vi "VGS Volume Project from RAW Volume.vi"() -> ()   [LabVIEW 2022 SP3, in "LV_VGS.lvlib"]
uses:
  LV_VGS.lvlib
  typedefs/3D Size (I32).ctl
  typedefs/3D Resolution (SGL).ctl
  RemoteControlClient/VGS_RemoteControlClient.lvclass
  Project/VGS_Project.lvclass
  VolumeDescriptor+File/VGS_VolumeDescriptor+File.lvclass
  VolumeDescriptor/VGS_VolumeDescriptor.lvclass
  ManufacturerInfo/VGS_ManufacturerInfo.lvclass
  ComponentInfo/VGS_ComponentInfo.lvclass
panel:
  out "Save Time, ms":u32=16563
  # "Original Volume Example rewritten in LabVIEW"
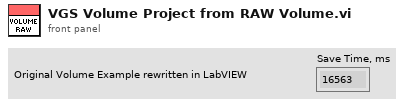
[diagram p1: front panel]
types:
  T1 = enum16{"big-endian, network order", "native, host order", "little-endian"}
  T2 = typedef "LV_VGS.lvlib/3D Resolution (SGL).ctl" = cluster{"X":sgl, "Y":sgl, "Z":sgl}
  T3 = typedef "LV_VGS.lvlib/3D Size (I32).ctl" = cluster{"X":i32, "Y":i32, "Z":i32}
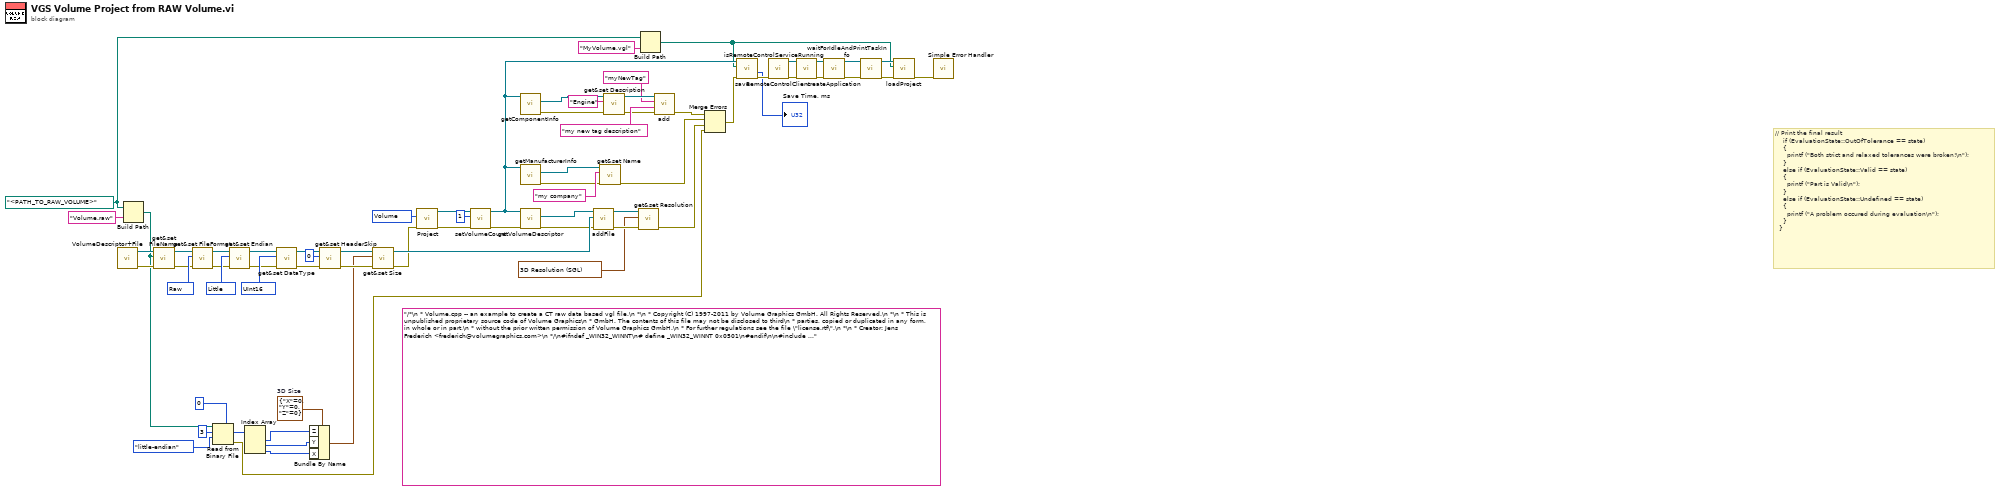
[diagram p0: block diagram]
diagram:
  w16 = 1448153088 items=["Volume"=1448153088, "Reconstruction"=1448153089] ("type")
  w7 = T3 {"X"=0, "Y"=0, "Z"=0}  # 3D Size
  w59 = 1448157378 items=["UInt8"=1448157376, "Int8"=1448157377, "UInt16"=1448157378, "Int16"=1448157379, "UInt32"=1448157380, "Int32"=1448157381, "Float"=1448157382, "Rgb8"=1448157383] ("DataType")
  w62 = 1448157440 items=["Little"=1448157440, "Big"=1448157441] ("Endian")
  w65 = 1448157312 items=["Raw"=1448157312, "Gzip"=1448157313, "Tiff"=1448157314, "Jpeg"=1448157315, "Bmp"=1448157316, "Bir"=1448157317, "Toshiba"=1448157318, "Shimadzu"=1448157319, "Pnm"=1448157320, "Jpeg2"=1448157321, "Yxlon"=1448157322, "Hdf"=1448157323, "Dicom"=1448157324, "Imtec"=1448157325, "Aracor"=1448157326, "Fhg"=1448157327] ("FileFormat")
  w18 = path "<PATH_TO_RAW_VOLUME>" ("replacementPattern")
  (unwired) "/*\n * Volume.cpp -- an example to create a CT raw data based vgl file.\n *\n * Copyright (C) 1997-2011 by Volume Graphics GmbH. All Rights Reserved.\n *\n * This is unpublished proprietary source code of Volume Graphics\n * GmbH. The contents of this file may not be disclosed to third\n * parties, copied or duplicated in any form, in whole or in part,\n * without the prior written permission of Volume Graphics GmbH.\n * For further regulations see the file \"license.rtf\".\n *\n * Creator: Jens Frederich <frederich@volumegraphics.com>\n */\n#ifndef _WIN32_WINNT\n# define _WIN32_WINNT 0x0501\n#endif\n\n#include <tchar.h>\n\n#include <vgs.project/project.h>\n\nusing namespace vgs::project;\nusing namespace vgs::project::volume;\n\nint _tmain (int argc, _TCHAR* argv[])\n{\n  Project* p = new Project (Project::Type::Volume);\n  assert (p != NULL);\n\n  // add single raw block file\n  {\n    VolumeDescriptor::File data;\n\n    data.setFileName   (\"D:/Volume Graphics/API TEST/vgs/data/engine.gz\");\n    data.setFileFormat (volume::FileFormat::Gzip);\n    data.setEndian     (volume::Endian::Little);\n    data.setDataType   (DataType::UInt8);\n    data.setHeaderSkip (0);\n    data.setSize       (Vector3<int> (256, 256, 110));\n    \n    p->setVolumeCount (1);\n    VolumeDescriptor* vd = p->getVolumeDescriptor (0);\n    assert (vd != NULL);\n\n    vd->addFile (data);\n  }\n\n  // add some meta data\n  {\n    ManufacturerInfo* mi = p->getManufacturerInfo ();\n    mi->setName (\"My company\");\n\n    ComponentInfo* ci = p->getComponentInfo ();\n    ci->setDescription (\"Engine\");\n\n    // add user defined tag\n    ci->add (\"myNewTag\", \"my new tag description\");\n\n    // add logo and preview\n    //p->setLogo    (\"c:/data/logo.png\");\n    //p->setPreview (\"c:/data/scene_preview.png\");\n  }\n\n  // create VG project\n  {\n    bool ok = true;\n\n    ok = p->save (std::string (\"D:/Volume Graphics/API TEST/vgs/data/my-first-volume1.vgl\"));\n    if (true != ok)\n    {\n      Error::ErrorCode err = Error::getLastError ();\n\t  printf(\"something is wrong, error code = %d\", err);\n      __debugbreak ();\n    }\n  }\n\n  // cleanup\n  if (p != NULL)\n  {\n    delete p;\n  }\n\n  return 0;\n}\n\n"
  # "// Print the final result\n    if (EvaluationState::OutOfTolerance == state)\n    {\n      printf (\"Both strict and relaxed tolerances were broken!\\n\");\n    }\n    else if (EvaluationState::Valid == state)\n    {\n      printf (\"Part is Valid\\n\");\n    }\n    else if (EvaluationState::Undefined == state)\n    {\n      printf (\"A problem occured during evaluation\\n\");\n    }\n  }"
  n1 = call "VolumeDescriptor+File.vi"() -> ("error out"=w67:errorcluster, "VGS_VolumeDescriptor+File out"=w69:refnum<class "VGS_VolumeDescriptor+File.lvclass">)  [unwired: 10 in]
  n2 = Build Path(base path=w18, name or relative path="Volume.raw") -> (appended path=w9:path)
  n3 = call "get&set FileName.vi"("error in (no error)"=w67, "FileName"=w9, "VGS_VolumeDescriptor+File in"=w69) -> ("error out"=w64:errorcluster, "VGS_VolumeDescriptor+File out"=w66:refnum<class "VGS_VolumeDescriptor+File.lvclass">)  [unwired: 6 in, 1 out]
  n4 = call "get&set FileFormat.vi"("error in (no error)"=w64, "FileFormat"=w65, "VGS_VolumeDescriptor+File in"=w66) -> ("error out"=w61:errorcluster, "VGS_VolumeDescriptor+File out"=w63:refnum<class "VGS_VolumeDescriptor+File.lvclass">)  [unwired: 6 in, 1 out]
  n5 = Read from Binary File(5:0, 9:T1."little-endian" ("byte order (0:big-endian, network order)"), 10:3 ("count (1)"), 11:w9) -> (0:w1:errorcluster, 2:w6:i32[])  [unwired: 2 in, 2 out]
  n6 = call "get&set Endian.vi"("error in (no error)"=w61, "Endian"=w62, "VGS_VolumeDescriptor+File in"=w63) -> ("error out"=w58:errorcluster, "VGS_VolumeDescriptor+File out"=w60:refnum<class "VGS_VolumeDescriptor+File.lvclass">)  [unwired: 6 in, 1 out]
  n7 = Index Array(array=w6) -> (element #1=w5:i32, element #2=w4:i32, element #3=w3:i32)  [unwired: 3 in]
  n8 = call "get&set DataType.vi"("error in (no error)"=w58, "DataType"=w59, "VGS_VolumeDescriptor+File in"=w60) -> ("error out"=w55:errorcluster, "VGS_VolumeDescriptor+File out"=w57:refnum<class "VGS_VolumeDescriptor+File.lvclass">)  [unwired: 6 in, 1 out]
  n9 = Bundle By Name(cluster=w7, "Z"=w5, "Y"=w4, "X"=w3) -> (w2:T3)
  n10 = call "get&set HeaderSkip.vi"("error in (no error)"=w55, "HeaderSkip"=0, "VGS_VolumeDescriptor+File in"=w57) -> ("error out"=w53:errorcluster, "VGS_VolumeDescriptor+File out"=w54:refnum<class "VGS_VolumeDescriptor+File.lvclass">)  [unwired: 6 in, 1 out]
  n11 = call "get&set Size.vi"("error in (no error)"=w53, "3D Size"=w2, "VGS_VolumeDescriptor+File in"=w54) -> ("error out"=w20:errorcluster, "VGS_VolumeDescriptor+File out"=w50:refnum<class "VGS_VolumeDescriptor+File.lvclass">)  [unwired: 6 in, 1 out]
  n12 = call "Project.vi"("error in (no error)"=w20, "type"=w16) -> ("error out"=w19:errorcluster, "VGS_Project out"=w52:refnum<class "VGS_Project.lvclass">)  [unwired: 8 in]
  n13 = call "setVolumeCount.vi"("error in (no error)"=w19, "VolumeCount"=u32 1, "VGS_Project in"=w52) -> ("error out"=w48:errorcluster, "VGS_Project out"=w38:refnum<class "VGS_Project.lvclass">)  [unwired: 7 in]
  n14 = call "getComponentInfo.vi"("VGS_Project in"=w38) -> ("error out"=w37:errorcluster, "VGS_ComponentInfo out"=w40:refnum<class "VGS_ComponentInfo.lvclass">)  [unwired: 8 in, 1 out]
  n15 = call "getManufacturerInfo.vi"("VGS_Project in"=w38) -> ("error out"=w35:errorcluster, "LV_VGS.lvlib:VGS_ManufacturerInfo.lvclass"=w39:refnum<class "VGS_ManufacturerInfo.lvclass">)  [unwired: 8 in, 1 out]
  n16 = call "getVolumeDescriptor.vi"("error in (no error)"=w48, "VGS_Project in"=w38) -> ("error out"=w47:errorcluster, "VGS_VolumeDescriptor out"=w49:refnum<class "VGS_VolumeDescriptor.lvclass">)  [unwired: 7 in, 1 out]
  n17 = call "addFile.vi"("error in (no error)"=w47, "LV_VGS.lvlib:VGS_VolumeDescriptor+File.lvclass"=w50, "VGS_VolumeDescriptor in"=w49) -> ("error out"=w15:errorcluster, "VGS_VolumeDescriptor out"=w13:refnum<class "VGS_VolumeDescriptor.lvclass">)  [unwired: 7 in]
  n18 = call "get&set Name.vi"("error in (no error)"=w35, "Name"="my company", "VGS_ManufacturerInfo in"=w39) -> ("error out"=w34:errorcluster)  [unwired: 6 in, 2 out]
  n19 = call "get&set Description.vi"("error in (no error)"=w37, "Description"="Engine", "VGS_ComponentInfo in"=w40) -> ("error out"=w36:errorcluster, "VGS_ComponentInfo out"=w44:refnum<class "VGS_ComponentInfo.lvclass">)  [unwired: 6 in, 1 out]
  n20 = call "get&set Resolution.vi"("error in (no error)"=w15, "3D Resolution"=T2 {"X"=0.0756, "Y"=0.0756, "Z"=0.0756}, "VGS_VolumeDescriptor in"=w13) -> ("error out"=w14:errorcluster)  [unwired: 6 in, 2 out]
  n21 = Build Path(base path=w18, name or relative path="MyVolume.vgl") -> (appended path=w21:path)
  n22 = call "add.vi"("error in (no error)"=w36, "description"="my new tag description", "tag"="myNewTag", "VGS_ComponentInfo in"=w44) -> ("error out"=w33:errorcluster)  [unwired: 6 in, 1 out]
  n23 = Merge Errors(w33, w34, w14, w1) -> (w32:errorcluster)
  n24 = call "save.vi"("error in (no error)"=w32, "Path"=w21, "VGS_Project in"=w38) -> ("error out"=w23:errorcluster, "Time, ms"=→"Save Time, ms":u32)  [unwired: 6 in, 1 out]
  n25 = call "RemoteControlClient.vi"("error in (no error)"=w23) -> ("error out"=w25:errorcluster, "VGS_RemoteControlClient out"=w24:refnum<class "VGS_RemoteControlClient.lvclass">)  [unwired: 9 in]
  n26 = call "isRemoteControlServiceRunning.vi"("error in (no error)"=w25, "VGS_RemoteControlClient in"=w24) -> ("error out"=w26:errorcluster, "VGS_RemoteControlClient out"=w27:refnum<class "VGS_RemoteControlClient.lvclass">)  [unwired: 7 in, 1 out]
  n27 = call "createApplication.vi"("error in (no error)"=w26, "VGS_RemoteControlClient in"=w27) -> ("error out"=w28:errorcluster, "VGS_RemoteControlClient out"=w31:refnum<class "VGS_RemoteControlClient.lvclass">)  [unwired: 8 in]
  n28 = call "waitForIdleAndPrintTaskInfo.vi"("error in (no error)"=w28, "VGS_RemoteControlClient in"=w31) -> ("error out"=w29:errorcluster, "VGS_RemoteControlClient out"=w30:refnum<class "VGS_RemoteControlClient.lvclass">)  [unwired: 8 in]
  n29 = call "loadProject.vi"("error in (no error)"=w29, "projectName"=w21, "VGS_RemoteControlClient in"=w30) -> ("error out"=w22:errorcluster)  [unwired: 7 in, 1 out]
  n30 = call <vilib>:"Simple Error Handler.vi"("error in (no error)"=w22) -> ()  [unwired: 4 in, 5 out]
